vi "VariableManagerTest.vi"() -> ()   [LabVIEW 2013]
uses:
  VariableManager.lvclass
  PackedLibraries/LuaEvaluatorAPI.lvlibp/API/t_Caching_Expression_Evaluator_Methods_Table.ctl
  Variable/Variable.lvclass
  API/VariableManagerAPI.lvlib
  PackedLibraries/LuaEvaluatorAPI.lvlibp
panel:
  in  "Tab Control":T1(tab)
  in  "EditIdx":bool
  in  "EditVar":bool
  in  "TestEventHandler":bool
  out "SequenceIndicesTable":string[][](table)
  in  "StopTest":bool
  in  "AddVar":bool
  in  "Variable Name":string
  in  "ReadVar":bool
  in  "DeleteVar":bool
  in  "DefaultValue":dbl
  in  "SequenceFunction":string
  in  "Sequence":bool
  in  "InformIgor":bool
  out "VariablesTable":string[][](table)
  in  "AddIdx":bool
  in  "Index Name":string
  in  "DeleteIdx":bool
  in  "Max":i32
  in  "Save":bool
  in  "Load":bool
  in  "Initialize":bool
  in  "expression/scriptlet":string="function LineRamp(f, Initial, Final)\n    return (1-f)*Initial + f*Final;\nend"
  in  "SequenceStepIn":i32
  out "VariableValues":cluster{"Name":string, "Value":dbl}[](array[cluster])
  in  "VariableManager":refnum<class "VariableManager.lvclass">
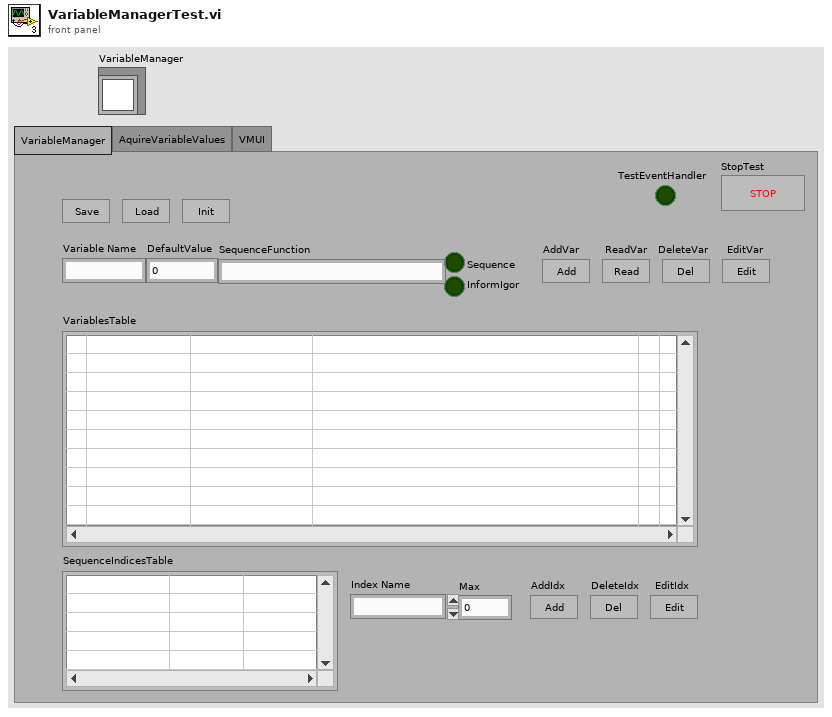
[diagram p1: front panel]
types:
  T1 = enum32{"VariableManager", "AquireVariableValues", "VMUI"}
  T2 = typedef "LuaEvaluatorAPI.lvlibp/t_Caching_Expression_Evaluator_Methods_Table.ctl" = enum16{"set", "get", "eval", "assign", "execute", "isvalid", "evaltable"}
  T3 = enum16{"open", "replace", "create", "open or create", "replace or create", "replace or create with confirmation"}
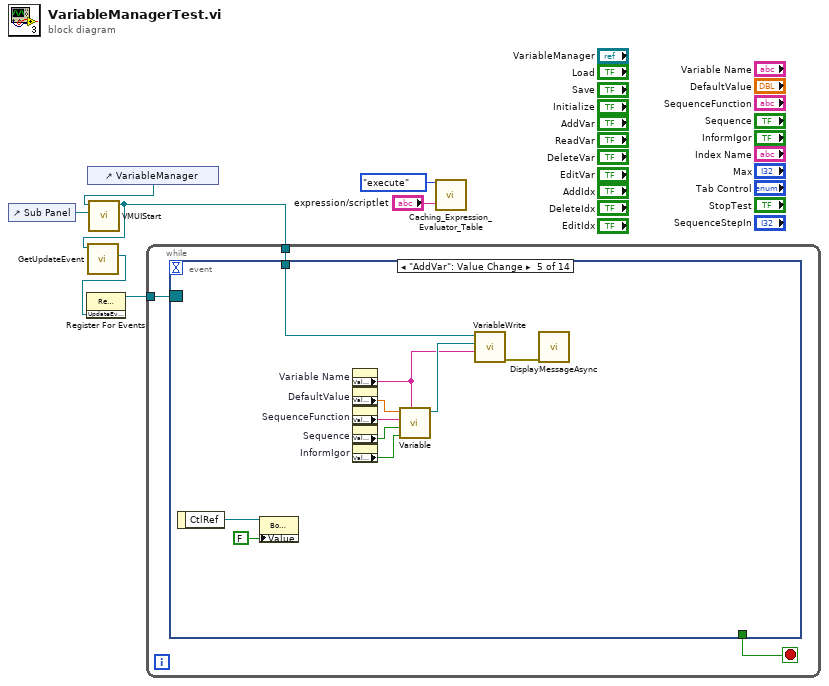
[diagram p0: block diagram]
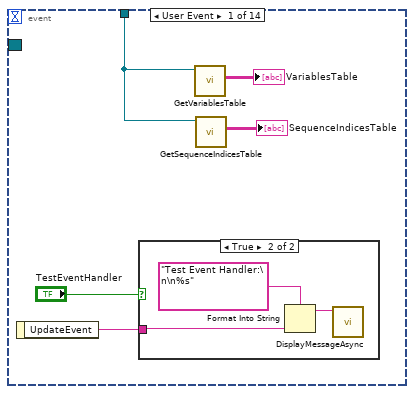
[diagram p2: hidden frame]
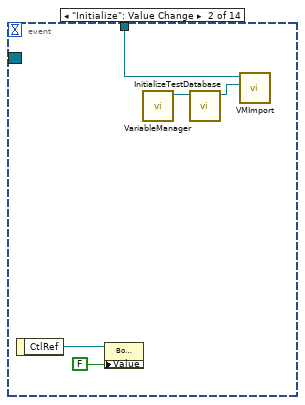
[diagram p4: hidden frame]
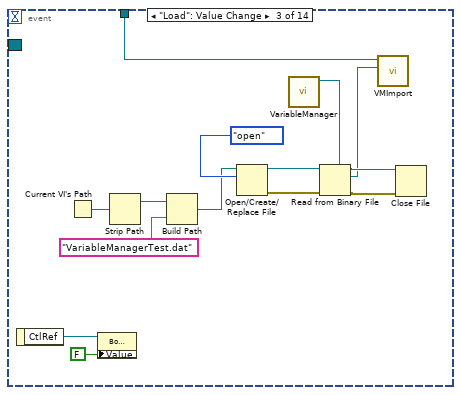
[diagram p5: hidden frame]
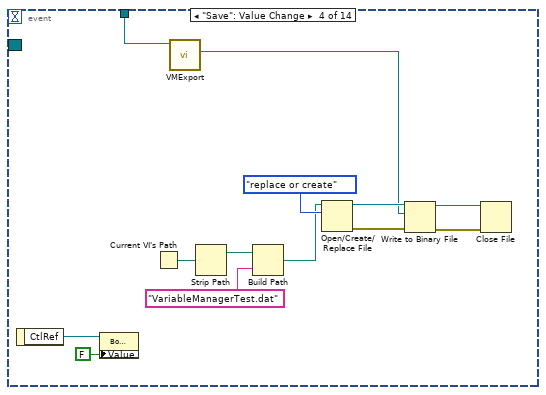
[diagram p6: hidden frame]
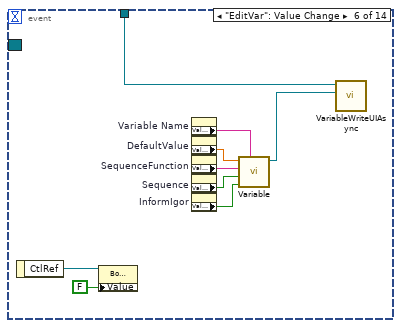
[diagram p7: hidden frame]
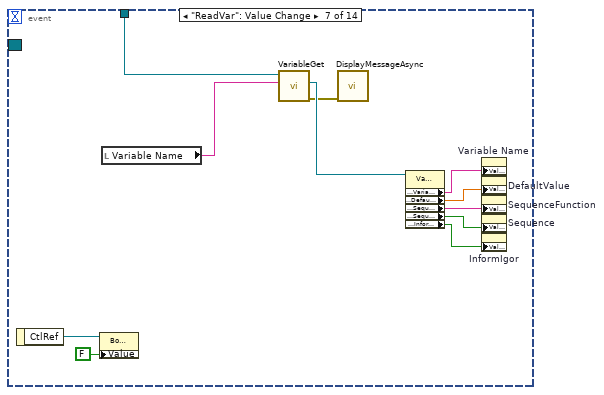
[diagram p8: hidden frame]
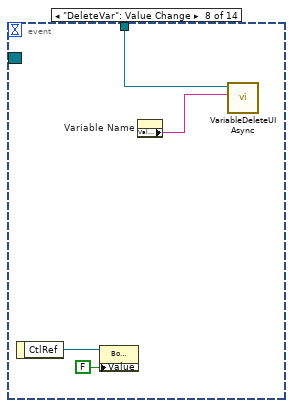
[diagram p9: hidden frame]
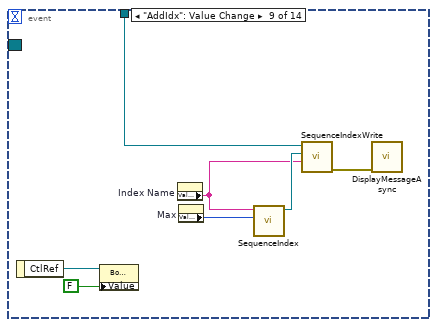
[diagram p10: hidden frame]
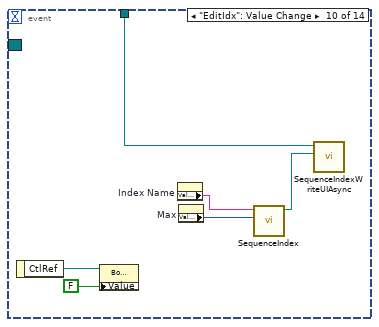
[diagram p11: hidden frame]
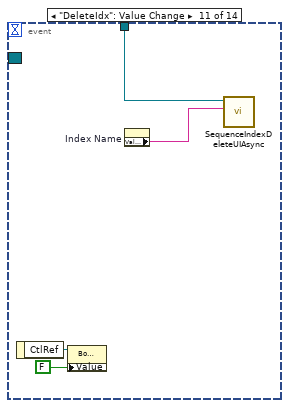
[diagram p12: hidden frame]
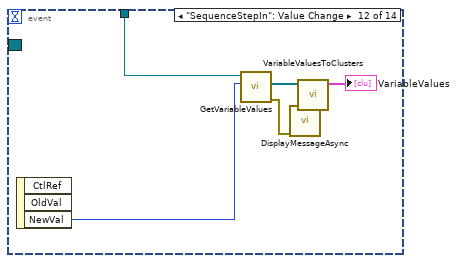
[diagram p13: hidden frame]
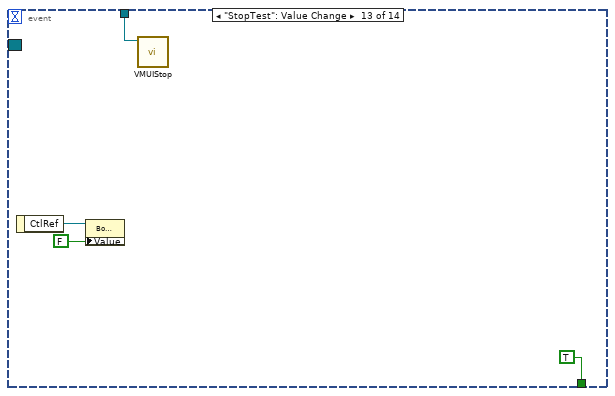
[diagram p14: hidden frame]
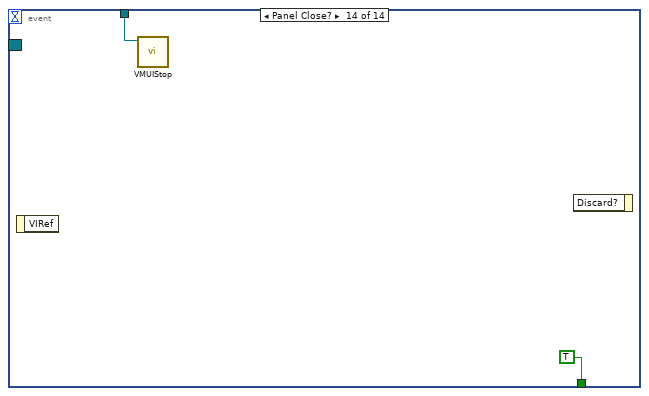
[diagram p15: hidden frame]
diagram:
  n1 = control-ref of="Sub Panel"() -> (w2:refnum<vi>)
  n2 = control-ref of="VariableManager"() -> (w5:refnum<vi>)
  n3 = call "VMUIStart.vi"("SubPanelRef"=w2, "VariableManagerRef in"=w5) -> ("VariableManagerRef out"=w4:refnum<vi>)  [unwired: 8 in, 1 out]
  n4 = call "GetUpdateEvent.vi"("VariableManagerRef in"=w4) -> ("UpdateEvent"=w6:refnum<user-event>)  [unwired: 8 in, 2 out]
  n5 = register-events(w6) -> (reference out=w3:refnum<event-registration>)  [unwired: 2 in, 1 out]
  n6 = while {
    tunnel: w4 -> [w10]
    tunnel: w3 -> [w9]
    stop <- w8 stop-if-true
    n7 = event shown="[4] \"AddVar\": Value Change" {
      selector: w9 -> [_ _ _ _ _ _ _ _ _ _ _ _ _ _]
      dyn-events: _ -> [_ _ _ _ _ _ _ _ _ _ _ _ _ _]
      timeout: _ -> [_ _ _ _ _ _ _ _ _ _ _ _ _ _]
      tunnel: w10 -> [w14 w20 w26 w39 w58 w62 w78 w82 w89 w93 w99 w106 w107 w111]
      tunnel: [_ _ _ _ _ _ _ _ _ _ _ _ TRUE TRUE] -> w8
      event User Event {
        n8 = event-data() -> ("UpdateEvent"=w15:string)  [unwired: 1 in]
        n9 = case shown="True" "TestEventHandler" {
          tunnel: w15 -> [_ w16]
          frame False {
          }
          frame True {
            n10 = Format Into String(format string="Test Event Handler:\n\n%s", w16) -> (resulting string=w18:string)  [unwired: 2 in, 1 out]
            n11 = call "DisplayMessageAsync.vi"("Message"=w18) -> ()  [unwired: 11 in]
          }
        }
        n12 = call "GetVariablesTable.vi"("VariableManagerRef in"=w14) -> ("VariableTable"=→"VariablesTable":string[][])  [unwired: 8 in, 2 out]
        n13 = call "GetSequenceIndicesTable.vi"("VariableManagerRef in"=w14) -> ("SequenceIndicesTable"=→"SequenceIndicesTable":string[][])  [unwired: 8 in, 2 out]
      }
      event "Initialize": Value Change {
        n14 = event-data() -> ("CtlRef"=w23:refnum<vi>)  [unwired: 1 in]
        n15 = property class="Bool (strict)"(reference=w23, "Value"=FALSE) -> ()  [unwired: 1 in, 2 out]
        n16 = call "VariableManager.vi"() -> ("VariableManager"=w21:refnum<class "VariableManager.lvclass">)  [unwired: 11 in]
        n17 = call-dynamic "InitializeTestDatabase.vi"("VariableManager in"=w21) -> ("VariableManager out"=w19:refnum<class "VariableManager.lvclass">)  [unwired: 9 in, 1 out]
        n18 = call "VMImport.vi"("VariableManager"=w19, "VariableManagerRef in"=w20) -> ()  [unwired: 8 in, 2 out]
      }
      event "Load": Value Change {
        n19 = event-data() -> ("CtlRef"=w36:refnum<vi>)  [unwired: 1 in]
        n20 = Current VI's Path() -> (path=w30:path)
        n21 = property class="Bool (strict)"(reference=w36, "Value"=FALSE) -> ()  [unwired: 1 in, 2 out]
        n22 = Strip Path(path=w30) -> (stripped path=w29:path)  [unwired: 1 out]
        n23 = Build Path(base path=w29, name or relative path="VariableManagerTest.dat") -> (appended path=w27:path)
        n24 = Open/Create/Replace File(file path (use dialog)=w27, operation (0:open)=T3."open") -> (refnum out=w34:refnum<file>, error out=w33:errorcluster)  [unwired: 4 in, 1 out]
        n25 = call "VariableManager.vi"() -> ("VariableManager"=w24:refnum<class "VariableManager.lvclass">)  [unwired: 11 in]
        n26 = Read from Binary File(5:w24, 8:w33, 11:w34) -> (0:w32:errorcluster, 2:w25:refnum<class "VariableManager.lvclass">, 3:w31:refnum<file>)  [unwired: 3 in, 1 out]
        n27 = call "VMImport.vi"("VariableManager"=w25, "VariableManagerRef in"=w26) -> ()  [unwired: 8 in, 2 out]
        n28 = Close File(refnum=w31, error in=w32) -> ()  [unwired: 2 out]
      }
      event "Save": Value Change {
        n29 = event-data() -> ("CtlRef"=w49:refnum<vi>)  [unwired: 1 in]
        n30 = property class="Bool (strict)"(reference=w49, "Value"=FALSE) -> ()  [unwired: 1 in, 2 out]
        n31 = Current VI's Path() -> (path=w43:path)
        n32 = call "VMExport.vi"("VariableManagerRef in"=w39) -> ("VariableManagerExportCopy"=w38:refnum<class "VariableManager.lvclass">)  [unwired: 8 in, 2 out]
        n33 = Strip Path(path=w43) -> (stripped path=w42:path)  [unwired: 1 out]
        n34 = Build Path(base path=w42, name or relative path="VariableManagerTest.dat") -> (appended path=w40:path)
        n35 = Open/Create/Replace File(file path (use dialog)=w40, operation (0:open)=T3."replace or create") -> (refnum out=w47:refnum<file>, error out=w45:errorcluster)  [unwired: 4 in, 1 out]
        n36 = Write to Binary File(file (use dialog)=w47, data=w38, error in=w45) -> (refnum out=w46:refnum<file>, error out=w44:errorcluster)  [unwired: 3 in, 1 out]
        n37 = Close File(refnum=w46, error in=w44) -> ()  [unwired: 2 out]
      }
      event "AddVar": Value Change {
        n38 = event-data() -> ("CtlRef"=w59:refnum<vi>)  [unwired: 1 in]
        n39 = property class="Bool (strict)"(reference=w59, "Value"=FALSE) -> ()  [unwired: 1 in, 2 out]
        n40 = property on="Variable Name" class="Str"() -> ("Value"=w55:string)  [unwired: 2 in, 2 out]
        n41 = property on="DefaultValue" class="DigNum (strict)"() -> ("Value"=w54:dbl)  [unwired: 2 in, 2 out]
        n42 = property on="SequenceFunction" class="Str"() -> ("Value"=w53:string)  [unwired: 2 in, 2 out]
        n43 = property on="Sequence" class="Bool (strict)"() -> ("Value"=w52:bool)  [unwired: 2 in, 2 out]
        n44 = property on="InformIgor" class="Bool (strict)"() -> ("Value"=w51:bool)  [unwired: 2 in, 2 out]
        n45 = call "Variable.vi"("VariableName"=w55, "InformIgor"=w51, "Sequence"=w52, "SequenceFunction"=w53, "DefaultValue"=w54) -> ("Variable"=w57:refnum<class "Variable.lvclass">)  [unwired: 6 in]
        n46 = call "VariableWrite.vi"("OriginalName"=w55, "Variable"=w57, "VariableManagerRef in"=w58) -> ("error out"=w56:errorcluster)  [unwired: 7 in, 1 out]
        n47 = call "DisplayMessageAsync.vi"("error in (no error)"=w56) -> ()  [unwired: 11 in]
      }
      event "EditVar": Value Change {
        n48 = event-data() -> ("CtlRef"=w68:refnum<vi>)  [unwired: 1 in]
        n49 = property class="Bool (strict)"(reference=w68, "Value"=FALSE) -> ()  [unwired: 1 in, 2 out]
        n50 = property on="Variable Name" class="Str"() -> ("Value"=w67:string)  [unwired: 2 in, 2 out]
        n51 = property on="DefaultValue" class="DigNum (strict)"() -> ("Value"=w66:dbl)  [unwired: 2 in, 2 out]
        n52 = property on="SequenceFunction" class="Str"() -> ("Value"=w65:string)  [unwired: 2 in, 2 out]
        n53 = property on="Sequence" class="Bool (strict)"() -> ("Value"=w64:bool)  [unwired: 2 in, 2 out]
        n54 = property on="InformIgor" class="Bool (strict)"() -> ("Value"=w63:bool)  [unwired: 2 in, 2 out]
        n55 = call "Variable.vi"("VariableName"=w67, "InformIgor"=w63, "Sequence"=w64, "SequenceFunction"=w65, "DefaultValue"=w66) -> ("Variable"=w61:refnum<class "Variable.lvclass">)  [unwired: 6 in]
        n56 = call "VariableWriteUIAsync.vi"("VariableFill"=w61, "VariableManagerRef in"=w62) -> ()  [unwired: 10 in]
      }
      event "ReadVar": Value Change {
        n57 = event-data() -> ("CtlRef"=w79:refnum<vi>)  [unwired: 1 in]
        n58 = property class="Bool (strict)"(reference=w79, "Value"=FALSE) -> ()  [unwired: 1 in, 2 out]
        n59 = local read "Variable Name"() -> (w77:string)
        n60 = call "VariableGet.vi"("VariableName"=w77, "VariableManagerRef in"=w78) -> ("error out"=w70:errorcluster, "Variable"=w76:refnum<class "Variable.lvclass">)  [unwired: 7 in, 1 out]
        n61 = call "DisplayMessageAsync.vi"("error in (no error)"=w70) -> ()  [unwired: 11 in]
        n62 = property class="Variable.lvclass"(reference=w76) -> ("Accessors:VariableName"=w75:string, "Accessors:DefaultValue"=w74:dbl, "Accessors:SequenceFunction"=w73:string, "Accessors:Sequence"=w72:bool, "Accessors:InformIgor"=w71:bool)  [unwired: 1 in, 2 out]
        n63 = property on="Variable Name" class="Str"("Value"=w75) -> ()  [unwired: 2 in, 2 out]
        n64 = property on="DefaultValue" class="DigNum (strict)"("Value"=w74) -> ()  [unwired: 2 in, 2 out]
        n65 = property on="SequenceFunction" class="Str"("Value"=w73) -> ()  [unwired: 2 in, 2 out]
        n66 = property on="Sequence" class="Bool (strict)"("Value"=w72) -> ()  [unwired: 2 in, 2 out]
        n67 = property on="InformIgor" class="Bool (strict)"("Value"=w71) -> ()  [unwired: 2 in, 2 out]
      }
      event "DeleteVar": Value Change {
        n68 = event-data() -> ("CtlRef"=w83:refnum<vi>)  [unwired: 1 in]
        n69 = property class="Bool (strict)"(reference=w83, "Value"=FALSE) -> ()  [unwired: 1 in, 2 out]
        n70 = property on="Variable Name" class="Str"() -> ("Value"=w81:string)  [unwired: 2 in, 2 out]
        n71 = call "VariableDeleteUIAsync.vi"("VariableName"=w81, "VariableManagerRef in"=w82) -> ()  [unwired: 10 in]
      }
      event "AddIdx": Value Change {
        n72 = event-data() -> ("CtlRef"=w91:refnum<vi>)  [unwired: 1 in]
        n73 = property class="Bool (strict)"(reference=w91, "Value"=FALSE) -> ()  [unwired: 1 in, 2 out]
        n74 = property on="Index Name" class="Str"() -> ("Value"=w86:string)  [unwired: 2 in, 2 out]
        n75 = property on="Max" class="DigNum (strict)"() -> ("Value"=w85:i32)  [unwired: 2 in, 2 out]
        n76 = call "SequenceIndex.vi"("Steps"=w85, "SequenceIndexName"=w86) -> ("SequenceIndex"=w88:refnum<class "SequenceIndex.lvclass">)  [unwired: 9 in]
        n77 = call "SequenceIndexWrite.vi"("OriginalName"=w86, "SequenceIndex"=w88, "VariableManagerRef in"=w89) -> ("error out"=w87:errorcluster)  [unwired: 7 in, 1 out]
        n78 = call "DisplayMessageAsync.vi"("error in (no error)"=w87) -> ()  [unwired: 11 in]
      }
      event "EditIdx": Value Change {
        n79 = event-data() -> ("CtlRef"=w97:refnum<vi>)  [unwired: 1 in]
        n80 = property class="Bool (strict)"(reference=w97, "Value"=FALSE) -> ()  [unwired: 1 in, 2 out]
        n81 = property on="Index Name" class="Str"() -> ("Value"=w95:string)  [unwired: 2 in, 2 out]
        n82 = property on="Max" class="DigNum (strict)"() -> ("Value"=w94:i32)  [unwired: 2 in, 2 out]
        n83 = call "SequenceIndex.vi"("Steps"=w94, "SequenceIndexName"=w95) -> ("SequenceIndex"=w92:refnum<class "SequenceIndex.lvclass">)  [unwired: 9 in]
        n84 = call "SequenceIndexWriteUIAsync.vi"("SequenceIndexFill"=w92, "VariableManagerRef in"=w93) -> ()  [unwired: 10 in]
      }
      event "DeleteIdx": Value Change {
        n85 = event-data() -> ("CtlRef"=w100:refnum<vi>)  [unwired: 1 in]
        n86 = property class="Bool (strict)"(reference=w100, "Value"=FALSE) -> ()  [unwired: 1 in, 2 out]
        n87 = property on="Index Name" class="Str"() -> ("Value"=w98:string)  [unwired: 2 in, 2 out]
        n88 = call "SequenceIndexDeleteUIAsync.vi"("SequenceIndexName"=w98, "VariableManagerRef in"=w99) -> ()  [unwired: 10 in]
      }
      event "SequenceStepIn": Value Change {
        n89 = event-data() -> ("NewVal"=w105:i32)  [unwired: 1 in, 2 out]
        n90 = call "GetVariableValues.vi"("SequenceStep"=w105, "VariableManagerRef in"=w106) -> ("error out"=w103:errorcluster, "VariableValues"=w102:refnum<class "VariableValue.lvclass">[])  [unwired: 7 in, 1 out]
        n91 = call "DisplayMessageAsync.vi"("error in (no error)"=w103) -> ()  [unwired: 11 in]
        n92 = call "VariableValuesToClusters.vi"("VariableValues"=w102) -> ("VariableValueClusters"=→"VariableValues":cluster{"Name":string, "Value":dbl}[])  [unwired: 10 in]
      }
      event "StopTest": Value Change {
        n93 = event-data() -> ("CtlRef"=w109:refnum<vi>)  [unwired: 1 in]
        n94 = property class="Bool (strict)"(reference=w109, "Value"=FALSE) -> ()  [unwired: 1 in, 2 out]
        n95 = call "VMUIStop.vi"("VariableManagerRef in"=w107) -> ()  [unwired: 9 in, 2 out]
      }
      event Panel Close? {
        n96 = event-data() -> ()  [unwired: 1 in, 1 out]
        n97 = call "VMUIStop.vi"("VariableManagerRef in"=w111) -> ()  [unwired: 9 in, 2 out]
        n98 = event-data() -> ()  [unwired: 2 in, 1 out]
      }
    }
  }
  n99 = call "Caching_Expression_Evaluator_Table.vi"("method"=t_Caching_Expression_Evaluator_Methods_Table."execute", "expression/scriptlet"="expression/scriptlet") -> ()  [unwired: 11 in, 3 out]
